vi "GetSettings.vi"(8 "error in (no error)":errorcluster, 10 "SettingsToRetrieve":variant, 11 "PacificPowerSource in":refnum<class "PacificPowerSource.lvclass">) -> (0 "error out":errorcluster, 2 "RetrievedSettings":variant, 3 "PacificPowerSource Out":refnum<class "PacificPowerSource.lvclass">)   [LabVIEW 2018, in "AcPwrPlugins.lvlib" / "PacificPowerSource.lvclass"]
doc: "This VI retrieves a boolean status to see if the instrument can conduct measurements while the device is changing modes or turning off and on."
uses:
  PacificPowerSource.lvclass
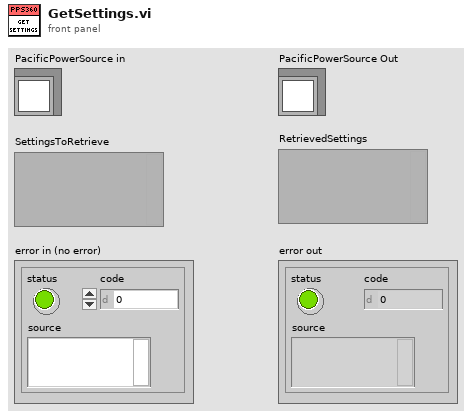
[diagram p1: front panel]
types:
  T1 = typedef "AcPwrPlugins.lvlib/PacificPowerSource.lvclass/DeviceSettings.ctl" = cluster{"MeasName":string, "Modules":cluster{"Handle":string, "Connected":bool, "Clear Device (F)":bool, "btnIdQuery":bool, "btnReset":bool, "Program #":cluster{"Phase B (Degrees)":i32, "Waveform A (1: Sine)":i32, "Voltage Level (Va)":dbl, "Program Number (0)":i32, "Voltage Level (Vb) ":dbl, "Form (3: Three)":u16, "Coupling  (0: Direct)":u16, "Frequency (45Hz)":dbl, "Current Limit (40A)":dbl, "Phase C (Degrees)":i32, "Voltage Level (Vc)":dbl, "Waveform B (1: Sine)":i32, "Waveform C (1: Sine)":i32}[], "Impedance Parameters (off, 0.00)":cluster{"State":bool, "Impedance":dbl}, "Transient Execution (F)":bool, "OutputEnabled":bool, "Source Range":cluster{"Frequency Minimum (45 Hz)":dbl, "Frequency Maximum (1200 Hz)":dbl, "Voltage Maximum (V)":dbl, "Voltage Minimum (V)":dbl, "Range Control (0: Auto)":u16, "Initial Voltage (0V)":u16, "Frequency Range (600Hz)":u16}, "Port Type":enum16{"GPIB", "Serial"}}[]}
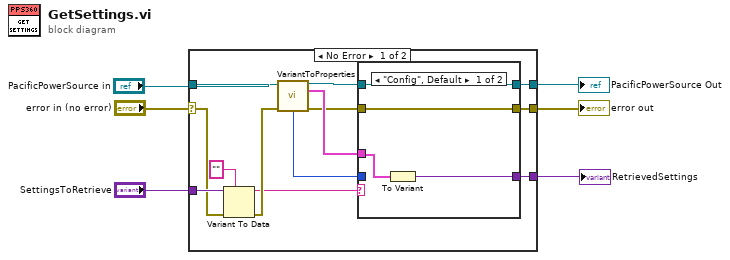
[diagram p0: block diagram]
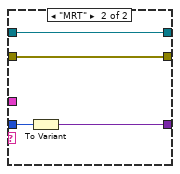
[diagram p2: hidden frame]
diagram:
  n1 = case shown="No Error" "error in (no error)" {
    selector: "error in (no error)" -> [w17 w29]
    tunnel: "PacificPowerSource in" -> [w19 w30]
    tunnel: [w10 w30] -> w3
    tunnel: [w8 w29] -> w2
    tunnel: "SettingsToRetrieve" -> [w18 w28]
    tunnel: [w14 w28] -> w1
    frame No Error {
      n2 = Variant To Data(error in=w17, type="", Variant=w18) -> (data=w13:string, error out=w16:errorcluster)
      n3 = call "VariantToProperties.vi"("PacificPowerSource in"=w19, "error in (no error)"=w16) -> ("PacificPowerSource out"=w11:refnum<class "PacificPowerSource.lvclass">, "Device(s)Settings"=w12:T1, "Measurement Refresh Time (ms)"=w7:u32, "error out"=w9:errorcluster)  [unwired: 7 in, 3 out]
      n4 = case shown="\"Config\", Default" w13 {
        tunnel: w12 -> [w22 _]
        tunnel: [w23 w26] -> w14
        tunnel: w7 -> [_ w27]
        tunnel: w11 -> [w21 w24]
        tunnel: [w21 w24] -> w10
        tunnel: w9 -> [w20 w25]
        tunnel: [w20 w25] -> w8
        frame "Config", Default {
          n5 = To Variant(anything=w22) -> (Variant=w23:variant)
        }
        frame "MRT" {
          n6 = To Variant(anything=w27) -> (Variant=w26:variant)
        }
      }
    }
    frame Error {
    }
  }
  "error out" <- w2
  "PacificPowerSource Out" <- w3
  "RetrievedSettings" <- w1
